vi "Protection.vi"() -> ()   [LabVIEW 2016]
uses:
  <vilib>/rvi/interface/nirviOpenFPGA/nirviOpenFPGA.xnode
  <vilib>/rvi/interface/nirviReadWriteControl/nirviReadWriteControl.xnode
  <vilib>/addons/Electrical Power/Basic/NI_EP_Basic.lvlib
  <vilib>/addons/Electrical Power/Basic/Measurement/RMS (N Channels).vi
  <vilib>/rvi/interface/nirviCloseFPGA/nirviCloseFPGA.xnode
  FPGA Bitfiles/IntelliRupter2_FPGATarget.lvbitx
  <vilib>/FPGAPlugInAG/cRIO-9039 (Sync)/niLvFpga_Open_cRIO-9039 (Sync).vi
  <vilib>/rvi/interface/common/dynamic/niFpgaDynamicAddResources.vi
  <vilib>/rvi/interface/Simulation/niFpgaSimulationCallBeginRW.vi
  <vilib>/rvi/errors/niLvFpgaAdjustHostInterfaceError.vi
  <vilib>/FPGAPlugInAG/Dynamic/niLvFpga_Close_Dynamic.vi
  <vilib>/addons/Electrical Power/Protection/Definite Time Delay/subVIs/fpga_Time Delay Cfg.ctl
  <vilib>/addons/Electrical Power/Protection/NI_EP_Protection_FPGA.lvlib
panel:
  in  "Manual trip":bool
  in  "Relay7":bool
  in  "Reclose?":bool
  in  "Recloser Settings":T1
  in  "time delay settings":T2
  out "VR error":i32
  out "VL error":i32
  in  "UV Reset level":dbl
  in  "Undervoltage \npick-up level":dbl
  in  "OC Reset level":dbl
  in  "Overcurrent\npick-up level":dbl
  out "I error":i32
  in  "stop":bool
  out "half cycle (samples)":i32=96
  out "basic calc interval":u16=38
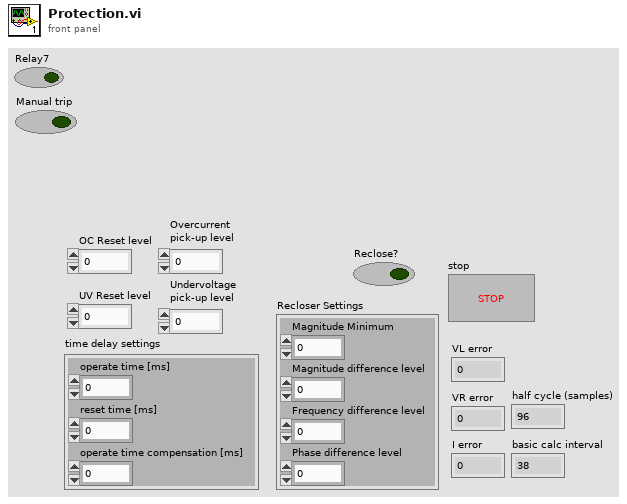
[diagram p1: front panel]
types:
  T1 = cluster{"Magnitude Minimum":dbl, "Magnitude difference level":dbl, "Frequency difference level":dbl, "Phase difference level":dbl}
  T2 = typedef "NI_EP_Protection_FPGA.lvlib/fpga_Time Delay Cfg.ctl" = cluster{"operate time [ms]":u32, "reset time [ms]":u32, "operate time compensation [ms]":u32}
  T3 = typedef "NI_EP_Protection_FPGA.lvlib/fpga_Timer Feedback Var.ctl" = cluster{"time elapsed":u32, "start time of trip counting":u32, "start time of reseting":u32}
  T4 = typedef "NI_EP_Protection_FPGA.lvlib/fpga_State.ctl" = enum16{"Idle", "Trip Counting", "Tripped", "Reset Counting"}
  T5 = cluster{"timing values out":T3, "status out":T4, "trip signal out":bool}
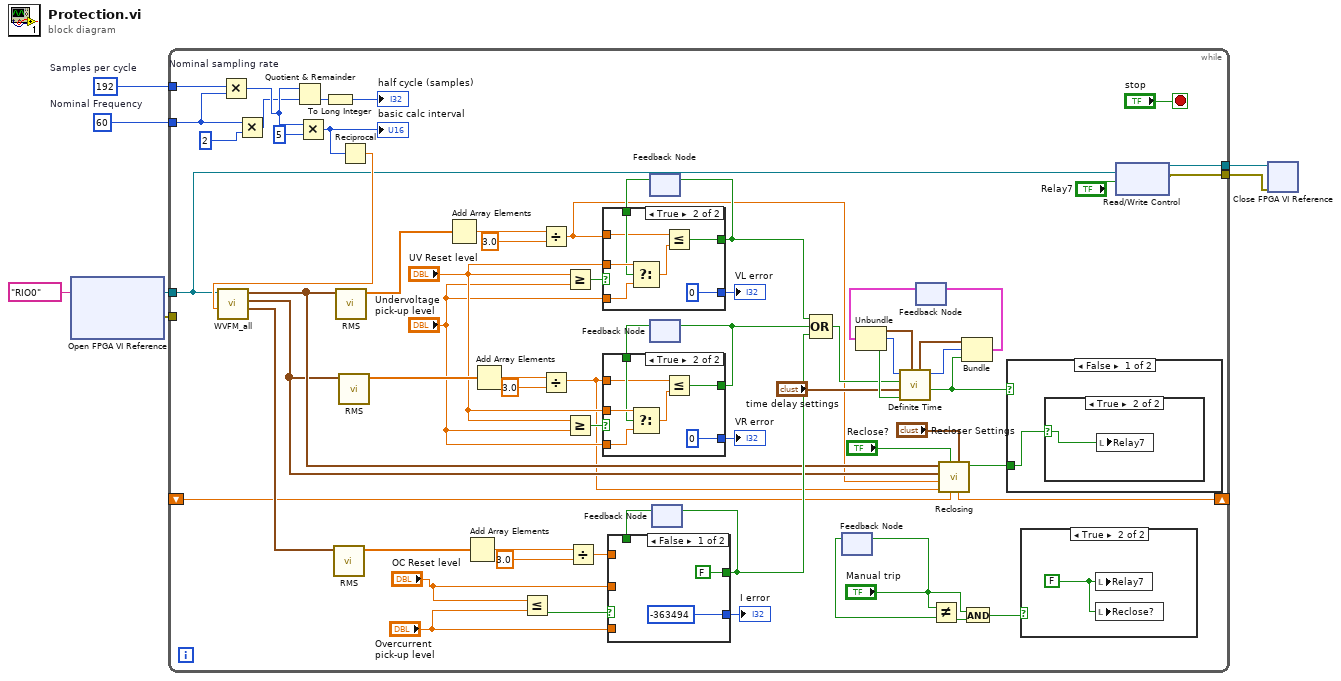
[diagram p0: block diagram]
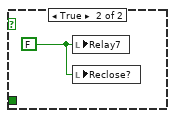
[diagram p3: hidden frame]
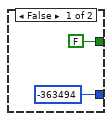
[diagram p5: hidden frame]
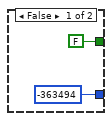
[diagram p6: hidden frame]
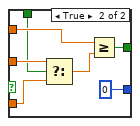
[diagram p7: hidden frame]
diagram:
  w3 = 192  # Samples per cycle
  w4 = 60  # Nominal Frequency
  n1 = xnode "Open FPGA VI Reference"("resource name"=tag "RIO0") -> ("FPGA VI Reference Out"=w7:refnum<k20>, "error out"=w6:errorcluster)  [unwired: 1 in]
  n2 = while {
    tunnel: w7 -> [w27]
    tunnel: w6 -> [_]
    tunnel: w4 -> [w65]
    tunnel: w3 -> [w64]
    shift-right: [w20] -> _
    shift-left: _ -> [w19]
    tunnel: [w18] -> w2
    tunnel: [w17] -> w1
    stop <- "stop" stop-if-true
    n3 = Multiply "Nominal sampling rate"(x=w64, y=w65) -> (x*y=w71:i32)
    n4 = Multiply(x=w65, y=2) -> (x*y=w67:i32)
    n5 = Quotient & Remainder(x=w71, y=w67) -> (floor(x/y)=w69:i32)  [unwired: 1 out]
    n6 = Multiply(x=w71, y=u16 5) -> (x*y=w72:i32)
    "basic calc interval" <- w72
    n7 = To Long Integer(number=w69) -> (32bit integer=→"half cycle (samples)":i32)
    n8 = Reciprocal(x=w72) -> (1/x=w62:dbl)
    n9 = call "WVFM_all.vi"("dt"=w62, "FPGA VI Reference"=w27) -> ("I array"=w61:waveform(sgl)[], "VR array"=w25:waveform(sgl)[], "VL array"=w26:waveform(sgl)[])  [unwired: 6 in]
    n10 = call-poly <vilib>:"RMS.vi"("waveforms"=w61) -> ("RMS values"=w58:dbl[])  [unwired: 9 in, 1 out]
    n11 = call-poly <vilib>:"RMS.vi"("waveforms"=w26) -> ("RMS values"=w51:dbl[])  [unwired: 9 in, 1 out]
    n12 = call-poly <vilib>:"RMS.vi"("waveforms"=w25) -> ("RMS values"=w42:dbl[])  [unwired: 9 in, 1 out]
    n13 = Add Array Elements(numeric array=w51) -> (sum=w50:dbl)
    n14 = Add Array Elements(numeric array=w58) -> (sum=w57:dbl)
    n15 = Add Array Elements(numeric array=w42) -> (sum=w45:dbl)
    n16 = Less Or Equal?(x="OC Reset level", y="Overcurrent\npick-up level") -> (x <= y?=w60:bool)
    n17 = Divide(x=w50, y=3.0) -> (x/y=w24:dbl)
    n18 = Divide(x=w45, y=3.0) -> (x/y=w23:dbl)
    n19 = Greater Or Equal?(x="UV Reset level", y="Undervoltage \npick-up level") -> (x >= y?=w54:bool)
    n20 = Greater Or Equal?(x="UV Reset level", y="Undervoltage \npick-up level") -> (x >= y?=w43:bool)
    n21 = Divide(x=w57, y=3.0 ("x")) -> (x/y=w56:dbl)
    n22 = feedback #1() -> (w52:bool)  [unwired: 1 in]
    n23 = case shown="True" w54 {
      tunnel: [FALSE w93] -> w39
      tunnel: [-363494 ("error") 0 ("error")] -> w48
      tunnel: "UV Reset level" -> [_ w91]
      tunnel: "Undervoltage \npick-up level" -> [_ w90]
      tunnel: w52 -> [_ w89]
      tunnel: w24 -> [_ w88]
      frame False {
      }
      frame True {
        n24 = Select(t=w91, s=w89, f=w90) -> (s? t:f=w94:dbl)
        n25 = Less Or Equal?(x=w88, y=w94) -> (x <= y?=w93:bool)
      }
    }
    "VL error" <- w48
    n26 = feedback-in #1(w39) -> ()
    n27 = feedback #2() -> (w44:bool)  [unwired: 1 in]
    n28 = case shown="True" w43 {
      tunnel: [FALSE w84] -> w38
      tunnel: [-363494 ("error") 0 ("error")] -> w47
      tunnel: "UV Reset level" -> [_ w82]
      tunnel: "Undervoltage \npick-up level" -> [_ w81]
      tunnel: w44 -> [_ w80]
      tunnel: w23 -> [_ w79]
      frame False {
      }
      frame True {
        n29 = Select(t=w82, s=w80, f=w81) -> (s? t:f=w85:dbl)
        n30 = Less Or Equal?(x=w79, y=w85) -> (x <= y?=w84:bool)
      }
    }
    "VR error" <- w47
    n31 = feedback-in #2(w38) -> ()
    n32 = feedback #3() -> (w53:bool)  [unwired: 1 in]
    n33 = case shown="False" w60 {
      tunnel: w56 -> [_ w103]
      tunnel: [-363494 ("error") 0 ("error")] -> w59
      tunnel: "OC Reset level" -> [_ w100]
      tunnel: "Overcurrent\npick-up level" -> [_ w99]
      tunnel: [FALSE ("Boolean") w98] -> w37
      tunnel: w53 -> [_ w97]
      frame False {
      }
      frame True {
        n34 = Select(t=w100, s=w97, f=w99) -> (s? t:f=w102:dbl)
        n35 = Greater Or Equal?(x=w103, y=w102) -> (x >= y?=w98:bool)
      }
    }
    "I error" <- w59
    n36 = feedback-in #3(w37) -> ()
    n37 = Compound Arithmetic op=OR(w39, w38, w37) -> (w29:bool)
    n38 = feedback #4() -> (w13:bool)  [unwired: 1 in]
    n39 = feedback-in #4("Manual trip") -> ()
    n40 = feedback #5() -> (w33:T5)  [unwired: 1 in]
    n41 = Unbundle(w33) -> ("timing values out"=w32:T3, "status out"=w31:T4, "trip signal out"=w30:bool)
    n42 = call "Definite Time.vi"("timing values in"=w32, "trip signal in"=w30, "time delay settings"="time delay settings", "pick-up signal? (F)"=w29, "status in"=w31) -> ("trip signal out"=w9:bool, "status out"=w35:T4, "timing values out"=w36:T3)  [unwired: 4 in]
    n43 = Not Equal?(x="Manual trip", y=w13) -> (x != y?=w12:bool)
    n44 = call "Reclosing.vi"("Recloser Settings"="Recloser Settings", "Counter In"=w19, "Reclose?"="Reclose?", "VR RMS avg"=w23, "VL RMS avg"=w24, "VR array"=w25, "VL array"=w26) -> ("Recloser action"=w8:bool, "Counter Out"=w20:dbl)  [unwired: 3 out]
    n45 = Bundle("timing values out"=w36, "status out"=w35, "trip signal out"=w9) -> (w34:T5)  [unwired: 1 in]
    n46 = feedback-in #5(w34) -> ()
    n47 = And(x="Manual trip", y=w12) -> (x .and. y?=w10:bool)
    n48 = case shown="False" w9 {
      tunnel: w8 -> [w73 _]
      frame False {
        n49 = case shown="True" w73 {
          selector: w73 -> [_ w74]
          frame False {
          }
          frame True {
            n50 = local write "Relay7"(w74) -> ()
          }
        }
      }
      frame True {
        w75 = FALSE ("Relay7")
        n51 = local write "Relay7"(w75) -> ()
        n52 = local write "Reclose?"(w75) -> ()
      }
    }
    n53 = case shown="True" w10 {
      frame False {
      }
      frame True {
        w76 = FALSE ("Relay7")
        n54 = local write "Relay7"(w76) -> ()
        n55 = local write "Reclose?"(w76) -> ()
      }
    }
    n56 = xnode "Read/Write Control"("FPGA VI Reference In"=w27, "Relay7"="Relay7") -> ("FPGA VI Reference Out"=w18:refnum<k20>, "error out"=w17:errorcluster)  [unwired: 1 in]
  }
  n57 = xnode "Close FPGA VI Reference"("FPGA VI Reference In"=w2, "error in"=w1) -> ()  [unwired: 1 out]
